vi "Parse RMC.vi"(8 "error in (no error)":errorcluster, 10 "Message":refnum<class "NMEA Message.lvclass">, 11 "nmea in":refnum<class "nmea.lvclass">) -> (0 "error out":errorcluster, 3 "nmea out":refnum<class "nmea.lvclass">)   [LabVIEW 2020, in "nmea.lvlib" / "nmea.lvclass"]
uses:
  nmea.lvclass
  message/NMEA Message.lvclass
  RMC Field.ctl
  nmea.lvclass/nmea.ctl
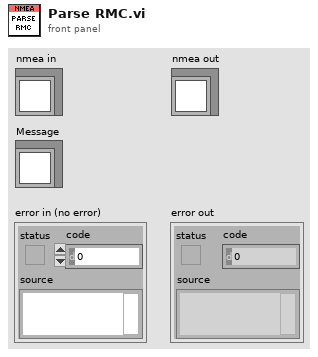
[diagram p1: front panel]
types:
  T1 = typedef "nmea.lvlib/nmea.lvclass/RMC Field.ctl" = enum16{"UTC Time", "Status", "Latitude", "N/S", "Longitude", "E/W", "Speed", "Course", "Date", "Mag Var", "Mag Var Dir", "Mode"}
  T2 = typedef "nmea.lvlib/nmea.lvclass/Ref Data.ctl" = cluster{"Latitude":dbl, "Longitude":dbl, "Time":T3, "Status":string, "Speed":dbl, "Course":dbl, "Mag Var":dbl, "Var Dir":string, "Mode":string, "Satellites":T4[], "Next Satellites":T4[], "Active PRNs":i32[], "Fix Type":T5, "DOP":T6, "Fix Mode":T7, "Altitude":dbl, "Geoid":dbl}
  T3 = typedef "LVDateTimeRec.ctl" = cluster{"fractional second":dbl, "second":i32, "minute":i32, "hour":i32, "day of month":i32, "month":i32, "year":i32, "day of week":i32, "day of year":i32, "DST":i32}
  T4 = typedef "nmea.lvlib/nmea.lvclass/Satellite.ctl" = cluster{"PRN":u8, "Channel":u8, "Elevation":u8, "Azimuth":u16, "SNR":u8, "Active":bool}
  T5 = typedef "nmea.lvlib/nmea.lvclass/Fix Type.ctl" = enum16{"N/A", "None", "2D", "3D"}
  T6 = typedef "nmea.lvlib/nmea.lvclass/DOP.ctl" = cluster{"P":dbl, "H":dbl, "V":dbl}
  T7 = typedef "nmea.lvlib/nmea.lvclass/Fix Mode.ctl" = enum16{"Manual", "Auto 2/3D"}
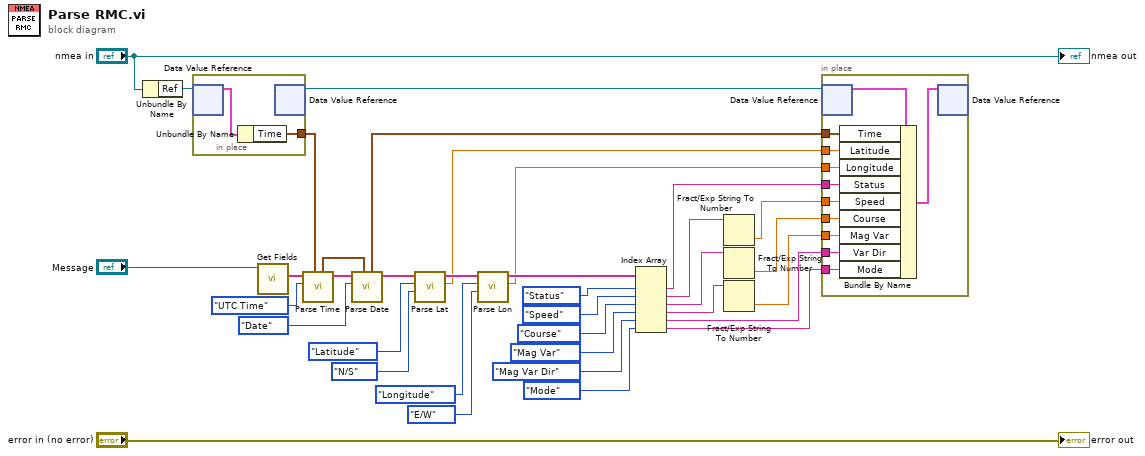
[diagram p0: block diagram]
diagram:
  n1 = Unbundle By Name("nmea in") -> ("Ref"=w25:refnum<data-value>)
  n2 = in-place {
    in-place-border: [w37] -> w24
    n3 = in-place-dvr #1(w25) -> (w38:T2)  [unwired: 1 out]
    n4 = Unbundle By Name(w38) -> ("Time"=w37:T3)
    n5 = in-place-dvr #1() -> (w10:refnum<data-value>)  [unwired: 1 in, 1 out]
  }
  n6 = call "Get Fields.vi"("NMEA Message in"="Message") -> ("Fields"=w34:string[])  [unwired: 8 in, 2 out]
  n7 = call "Parse Time.vi"("Time In"=w24, "Time Index"=RMC_Field."UTC Time" ("RMC Field"), "Fields In"=w34) -> ("Fields"=w23:string[], "Time"=w20:T3)  [unwired: 7 in]
  n8 = call "Parse Date.vi"("Time In"=w20, "Date Index"=RMC_Field."Date" ("RMC Field"), "Fields In"=w23) -> ("Fields"=w21:string[], "Time"=w9:T3)  [unwired: 7 in]
  n9 = call "Parse Lat.vi"("N/S Index"=RMC_Field."N/S" ("RMC Field"), "Latitude Index"=RMC_Field."Latitude" ("RMC Field"), "Fields In"=w21) -> ("Latitude"=w8:dbl, "Fields"=w29:string[])  [unwired: 7 in]
  n10 = call "Parse Lon.vi"("E/W Index"=RMC_Field."E/W" ("RMC Field"), "Longitude Index"=RMC_Field."Longitude" ("RMC Field"), "Fields In"=w29) -> ("Longitude"=w7:dbl, "Fields"=w19:string[])  [unwired: 7 in]
  n11 = Index Array(array=w19, index #1=RMC_Field."Status" ("RMC Field"), index #2=RMC_Field."Speed" ("RMC Field"), index #3=RMC_Field."Course" ("RMC Field"), index #4=RMC_Field."Mag Var" ("RMC Field"), index #5=RMC_Field."Mag Var Dir" ("RMC Field"), index #6=RMC_Field."Mode" ("RMC Field")) -> (element #1=w6:string, element #2=w13:string, element #3=w12:string, element #4=w11:string, element #5=w2:string, element #6=w1:string)
  n12 = Fract/Exp String To Number(string=w13) -> (number=w5:dbl)  [unwired: 3 in, 1 out]
  n13 = Fract/Exp String To Number(string=w12) -> (number=w4:dbl)  [unwired: 3 in, 1 out]
  n14 = Fract/Exp String To Number(string=w11) -> (number=w3:dbl)  [unwired: 3 in, 1 out]
  n15 = in-place {
    in-place-border: w9 -> [w48]
    in-place-border: w8 -> [w47]
    in-place-border: w7 -> [w46]
    in-place-border: w6 -> [w45]
    in-place-border: w5 -> [w44]
    in-place-border: w4 -> [w43]
    in-place-border: w3 -> [w42]
    in-place-border: w2 -> [w41]
    in-place-border: w1 -> [w40]
    n16 = in-place-dvr #2(w10) -> (w49:T2)  [unwired: 1 out]
    n17 = Bundle By Name(cluster=w49, "Time"=w48, "Latitude"=w47, "Longitude"=w46, "Status"=w45, "Speed"=w44, "Course"=w43, "Mag Var"=w42, "Var Dir"=w41, "Mode"=w40) -> (w39:T2)
    n18 = in-place-dvr #2(w39) -> ()  [unwired: 2 out]
  }
  "error out" <- "error in (no error)"
  "nmea out" <- "nmea in"
